vi "Remove Notifier.vi"(8 "error in (no error)":errorcluster, 10 "ID In":variant, 11 "Simple Map Notifier Controller in":refnum<class "Simple Map SEQ I64 Notifier Controller.lvclass">) -> (0 "error out":errorcluster, 3 "Simple Map Notifier Controller out":refnum<class "Simple Map SEQ I64 Notifier Controller.lvclass">)   [LabVIEW 2022 SP3, in "Simple Map SEQ I64 Notifier Controller.lvclass"]
uses:
  Simple Map SEQ I64 Notifier Controller.lvclass
  Simple Map SEQ I64 Notifier Controller.lvclass/Simple Map SEQ I64 Notifier Controller.ctl
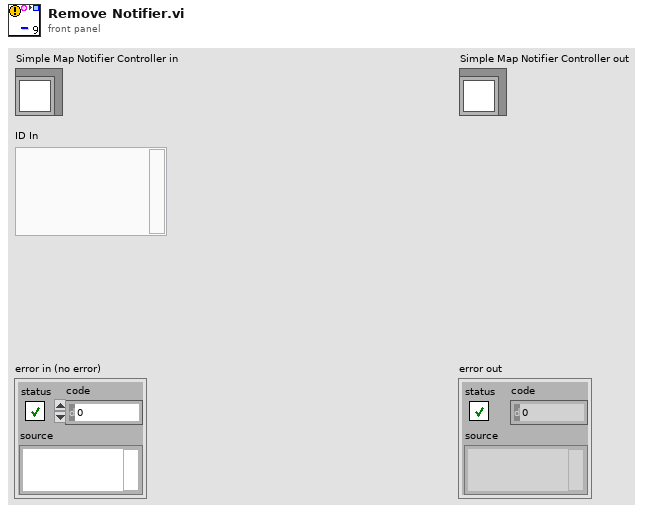
[diagram p1: front panel]
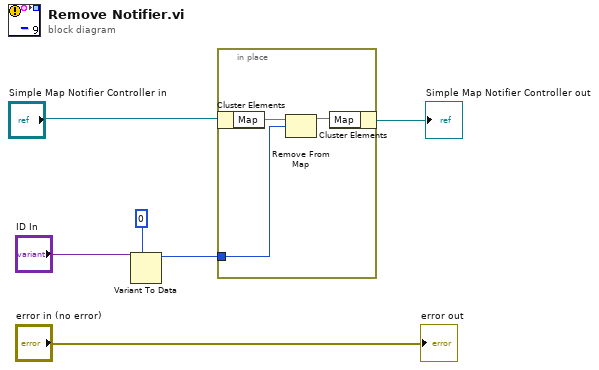
[diagram p0: block diagram]
diagram:
  n1 = Variant To Data(type=i64 0, Variant="ID In") -> (data=w5:i64)  [unwired: 1 in, 1 out]
  n2 = in-place {
    in-place-border: w5 -> [w7]
    n3 = in-place-cluster #1("Simple Map Notifier Controller in") -> ("Map"=w9:map{i64, refnum<class "Notifier.lvclass">})
    n4 = Remove From Map(10:w7, 11:w9) -> (3:w8:map{i64, refnum<class "Notifier.lvclass">})  [unwired: 2 out]
    n5 = in-place-cluster #1("Map"=w8) -> (→"Simple Map Notifier Controller out":refnum<class "Simple Map SEQ I64 Notifier Controller.lvclass">)
  }
  "error out" <- "error in (no error)"
